vi "Periodic Tasks.vi"(8 "error in":errorcluster) -> ()   [LabVIEW 2016]
doc: "This VI runs in parallel to other tasks. It can contain as many user-defined periodic loops as you need. These can carry out PID or other sorts of timed response."
uses:
  <vilib>/Rock Robotics/WPI/Utilities/WPI_GetSetVariantRefNum.vi
  drive diraction.vi
  <vilib>/Rock Robotics/Network Tables/NT Write Boolean.vi
panel:
  out "rad":bool
  in  "pull":bool
  in  "push":bool
  in  "fire":bool
  in  "gear diraction":bool
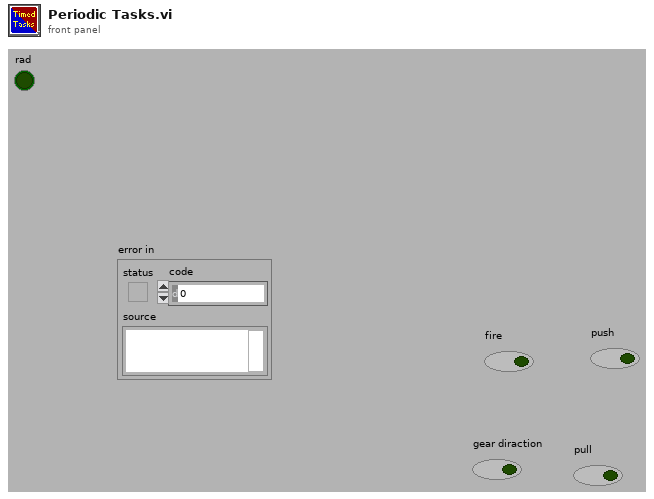
[diagram p1: front panel]
types:
  T1 = typedef "WPI_JoystickDevRef.ctl" = cluster{"Device":T2}
  T2 = typedef "WPI_JoystickDeviceEnum.ctl" = enum16{"USB 0", "USB 1", "USB 2", "USB 3", "USB 4", "USB 5"}
  T3 = cluster{"Buttons[0]":bool, "Buttons[1]":bool, "Buttons[2]":bool, "Buttons[3]":bool, "Buttons[4]":bool, "Buttons[5]":bool, "Buttons[6]":bool, "Buttons[7]":bool, "Buttons[8]":bool}
  T4 = typedef "WPI_MotorControlDeviceRef.ctl" = cluster{"DeviceStatus":errorcluster, "Type":T5, "PWM":cluster{"PWM Channel":T6, "DeadBand":T7}, "CAN":cluster{"Device Number":u8, "SetOutput VI Ref":variant, "GetOutput VI Ref":variant, "Enable VI Ref":variant, "Disable VI Ref":variant, "Data":variant}, "Invert":bool}
  T5 = typedef "WPI_MotorControlType.ctl" = enum16{"PWM", "CAN"}
  T6 = typedef "FPGA_DIOPWMChannel.ctl" = enum8{"PWM 0", "PWM 1", "PWM 2", "PWM 3", "PWM 4", "PWM 5", "PWM 6", "PWM 7", "PWM 8", "PWM 9", "PWM MXP 0", "PWM MXP 1", "PWM MXP 2", "PWM MXP 3", "PWM MXP 4", "PWM MXP 5", "PWM MXP 6", "PWM MXP 7", "PWM MXP 8", "PWM MXP 9", "Invalid"}
  T7 = typedef "WPI_PWMDeadband.ctl" = cluster{"Name":string, "maxPositivePwm":i32, "minPositivePwm":i32, "centerPwm":i32, "maxNegativePwm":i32, "minNegativePwm":i32, "angularRange":u16}
  T8 = typedef "WPI_DigitalInputDevRef.ctl" = cluster{"DevStatus":errorcluster, "DIO Channel":T9}
  T9 = typedef "FPGA_DIOChannel.ctl" = enum8{"DIO 0", "DIO 1", "DIO 2", "DIO 3", "DIO 4", "DIO 5", "DIO 6", "DIO 7", "DIO 8", "DIO 9", "DIO MXP 0", "DIO MXP 1", "DIO MXP 2", "DIO MXP 3", "DIO MXP 4", "DIO MXP 5", "DIO MXP 6", "DIO MXP 7", "DIO MXP 8", "DIO MXP 9", "DIO MXP 10", "DIO MXP 11", "DIO MXP 12", "DIO MXP 13", "DIO MXP 14", "DIO MXP 15", "SPI Port CS1", "SPI Port CS2", "SPI Port CS3", "SPI Port MISO", "SPI Port MOSI", "Invalid"}
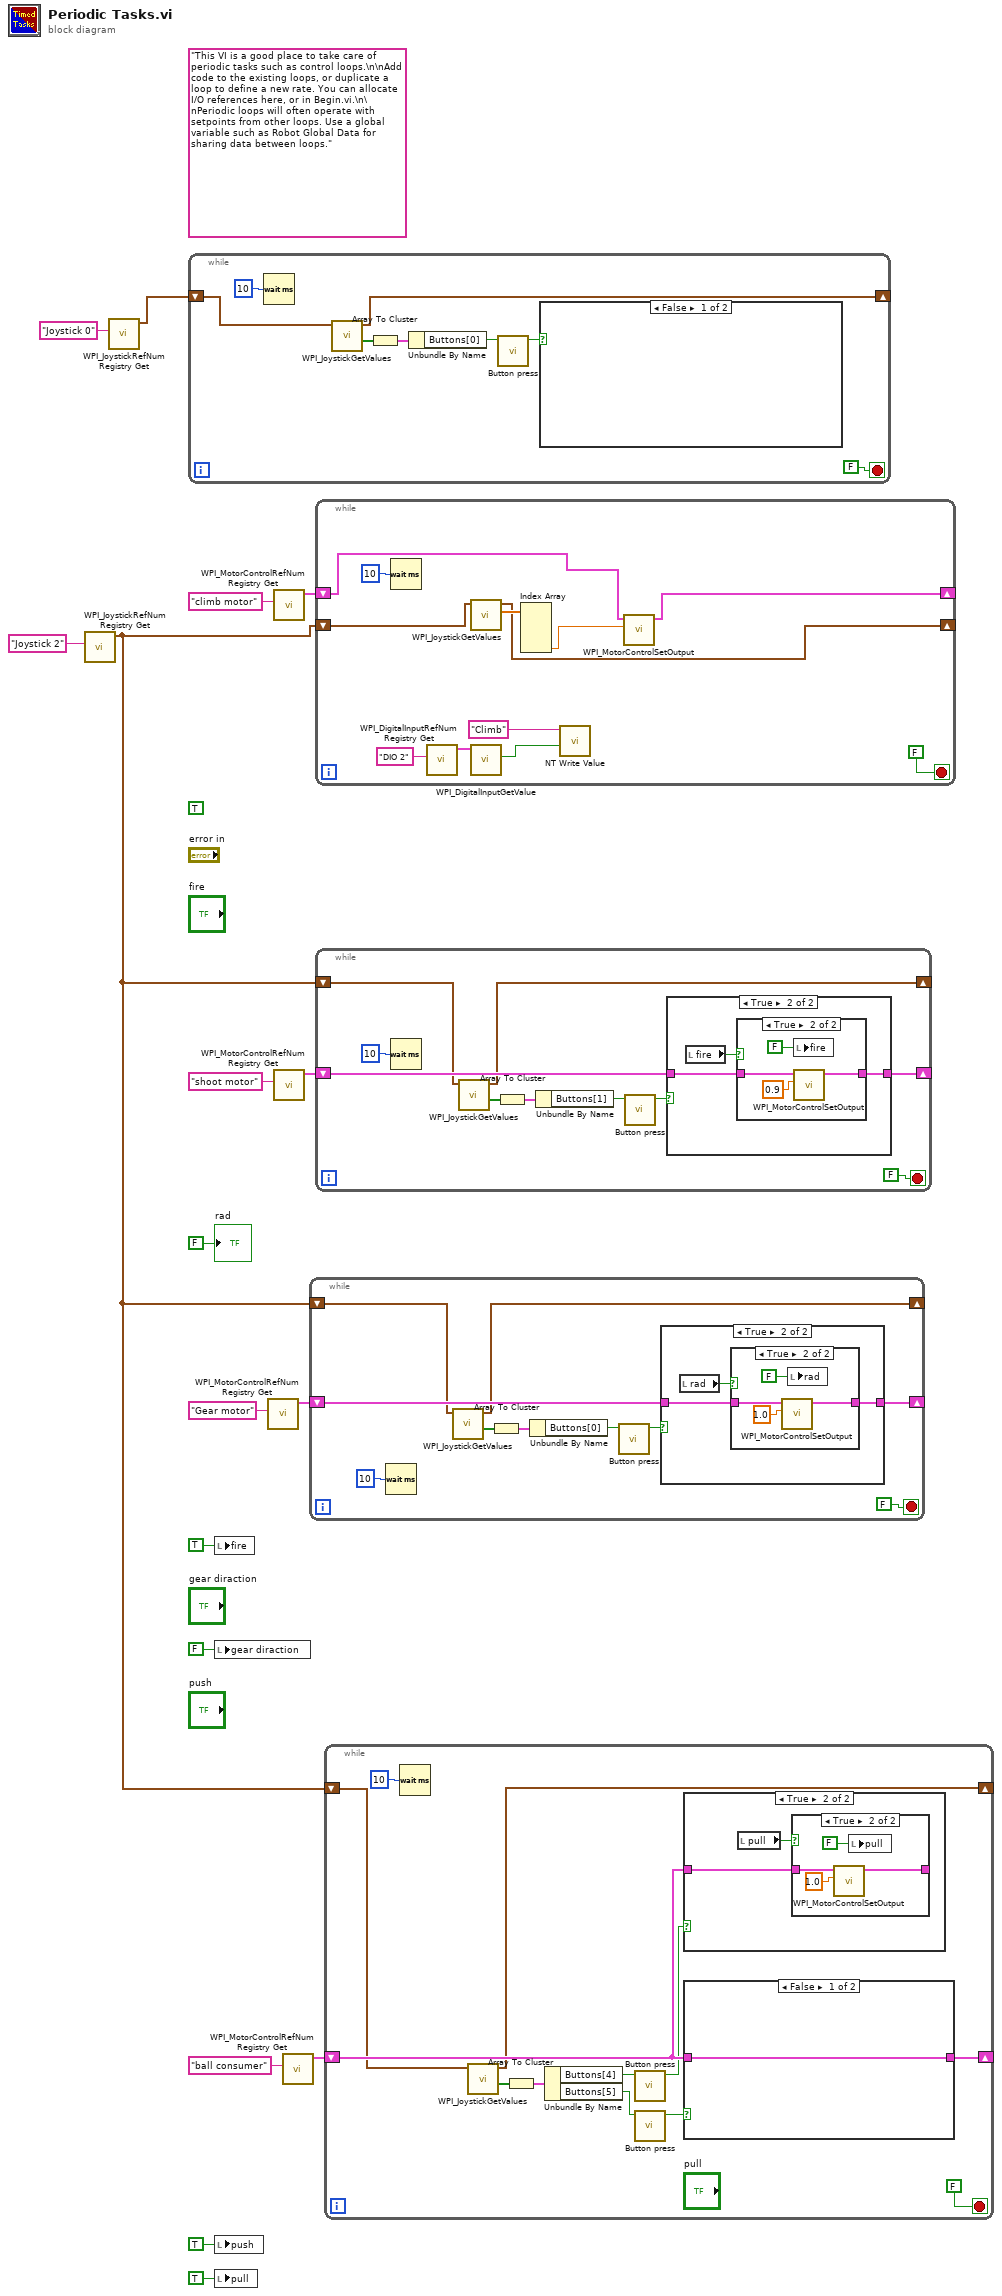
[diagram p0: block diagram]
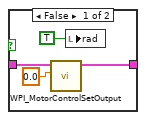
[diagram p3: hidden frame]
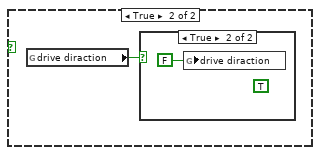
[diagram p4: hidden frame]
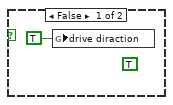
[diagram p5: hidden frame]
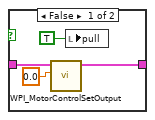
[diagram p7: hidden frame]
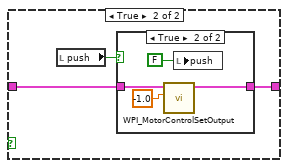
[diagram p8: hidden frame]
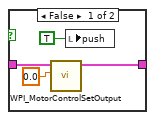
[diagram p9: hidden frame]
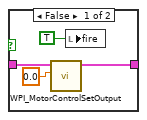
[diagram p11: hidden frame]
diagram:
  (unwired) TRUE ("fire")
  (unwired) "This VI is a good place to take care of periodic tasks such as control loops.\n\nAdd code to the existing loops, or duplicate a loop to define a new rate. You can allocate I/O references here, or in Begin.vi.\n\nPeriodic loops will often operate with setpoints from other loops. Use a global variable such as Robot Global Data for sharing data between loops."
  n1 = call <vilib>:"WPI_JoystickRefNum Registry Get.vi"("refnum name"="Joystick 2") -> ("JoystickDevRef"=w1:T1)  [unwired: 1 in, 9 out]
  n2 = call <vilib>:"WPI_JoystickRefNum Registry Get.vi"("refnum name"="Joystick 0") -> ("JoystickDevRef"=w3:T1)  [unwired: 1 in, 9 out]
  n3 = while {
    shift-right: [w18] -> _
    shift-left: w3 -> [w19]
    stop <- FALSE stop-if-true
    n4 = Wait (ms)(milliseconds to wait=u32 10) -> ()  [unwired: 1 out]
    n5 = call <vilib>:"WPI_JoystickGetValues.vi"("JoystickDevRef"=w19) -> ("Buttons"=w24:bool[], "JoystickDevRef"=w18:T1)  [unwired: 6 in, 3 out]
    n6 = Array To Cluster(array=w24) -> (cluster=w23:T3)
    n7 = Unbundle By Name(w23) -> ("Buttons[0]"=w21:bool)
    n8 = call "Button press.vi"("Boolean"=w21) -> ("Boolean 2"=w20:bool)  [unwired: 10 in]
    n9 = case shown="False" w20 {
      frame False {
      }
      frame True {
        n10 = global read "drive diraction.vi" "drive diraction"() -> (w26:bool)
        n11 = case shown="True" w26 {
          frame False {
            (unwired) TRUE ("fire")
            n12 = global write "drive diraction.vi" "drive diraction"(TRUE ("drive diraction")) -> ()
          }
          frame True {
            (unwired) TRUE ("fire")
            n13 = global write "drive diraction.vi" "drive diraction"(FALSE ("drive diraction")) -> ()
          }
        }
      }
    }
  }
  n14 = local write "fire"(TRUE ("fire")) -> ()
  n15 = local write "gear diraction"(FALSE ("gear diraction")) -> ()
  n16 = local write "push"(TRUE ("push")) -> ()
  n17 = local write "pull"(TRUE ("pull")) -> ()
  n18 = call <vilib>:"WPI_MotorControlRefNum Registry Get.vi"("refnum name"="Gear motor") -> ("MotorControlDevRef"=w6:T4)  [unwired: 9 in, 1 out]
  n19 = call <vilib>:"WPI_MotorControlRefNum Registry Get.vi"("refnum name"="climb motor") -> ("MotorControlDevRef"=w16:T4)  [unwired: 9 in, 1 out]
  n20 = call <vilib>:"WPI_MotorControlRefNum Registry Get.vi"("refnum name"="shoot motor") -> ("MotorControlDevRef"=w15:T4)  [unwired: 9 in, 1 out]
  n21 = call <vilib>:"WPI_MotorControlRefNum Registry Get.vi"("refnum name"="ball consumer") -> ("MotorControlDevRef"=w12:T4)  [unwired: 9 in, 1 out]
  n22 = while {
    shift-right: [w34] -> _
    shift-left: w6 -> [w35]
    shift-right: [w30] -> _
    shift-left: w1 -> [w31]
    stop <- FALSE stop-if-true
    n23 = Wait (ms)(milliseconds to wait=u32 10) -> ()  [unwired: 1 out]
    n24 = call <vilib>:"WPI_JoystickGetValues.vi"("JoystickDevRef"=w31) -> ("Buttons"=w36:bool[], "JoystickDevRef"=w30:T1)  [unwired: 6 in, 3 out]
    n25 = Array To Cluster(array=w36) -> (cluster=w37:T3)
    n26 = Unbundle By Name(w37) -> ("Buttons[0]"=w32:bool)
    n27 = call "Button press.vi"("Boolean"=w32) -> ("Boolean 2"=w33:bool)  [unwired: 10 in]
    n28 = case shown="True" w33 {
      tunnel: w35 -> [w39 w40]
      tunnel: [w39 w41] -> w34
      frame False {
      }
      frame True {
        n29 = local read "rad"() -> (w42:bool)
        n30 = case shown="True" w42 {
          tunnel: [w44 w49] -> w41
          tunnel: w40 -> [w45 w48]
          frame False {
            n31 = call <vilib>:"WPI_MotorControlSetOutput.vi"("Output"=0.0, "MotorControlDevRef"=w45) -> ("MotorControlDevRef"=w44:T4)  [unwired: 7 in, 2 out]
            n32 = local write "rad"(TRUE ("rad")) -> ()
          }
          frame True {
            n33 = call <vilib>:"WPI_MotorControlSetOutput.vi"("Output"=1.0, "MotorControlDevRef"=w48) -> ("MotorControlDevRef"=w49:T4)  [unwired: 7 in, 2 out]
            n34 = local write "rad"(FALSE ("rad")) -> ()
          }
        }
      }
    }
  }
  n35 = while {
    shift-right: [w54] -> _
    shift-left: w16 -> [w55]
    shift-right: [w51] -> _
    shift-left: w1 -> [w52]
    stop <- FALSE stop-if-true
    n36 = Wait (ms)(milliseconds to wait=u32 10) -> ()  [unwired: 1 out]
    n37 = call <vilib>:"WPI_DigitalInputRefNum Registry Get.vi"("refnum name"="DIO 2") -> ("DigitalInputDevRef"=w59:T8)  [unwired: 9 in, 1 out]
    n38 = call <vilib>:"WPI_JoystickGetValues.vi"("JoystickDevRef"=w52) -> ("Axes"=w56:dbl[], "JoystickDevRef"=w51:T1)  [unwired: 6 in, 3 out]
    n39 = call <vilib>:"WPI_DigitalInputGetValue.vi"("DigitalInputDevRef"=w59) -> ("Value"=w58:bool)  [unwired: 8 in, 2 out]
    n40 = Index Array(array=w56) -> (element #4=w53:dbl)  [unwired: 4 in, 3 out]
    n41 = call-poly <vilib>:"NT Write Value.vi"("Boolean"=w58, "Name"="Climb") -> ()  [unwired: 9 in, 1 out]
    n42 = call <vilib>:"WPI_MotorControlSetOutput.vi"("Output"=w53, "MotorControlDevRef"=w55) -> ("MotorControlDevRef"=w54:T4)  [unwired: 7 in, 2 out]
  }
  n43 = while {
    shift-right: [w69] -> _
    shift-left: w15 -> [w68]
    shift-right: [w63] -> _
    shift-left: w1 -> [w64]
    stop <- FALSE stop-if-true
    n44 = Wait (ms)(milliseconds to wait=u32 10) -> ()  [unwired: 1 out]
    n45 = call <vilib>:"WPI_JoystickGetValues.vi"("JoystickDevRef"=w64) -> ("Buttons"=w71:bool[], "JoystickDevRef"=w63:T1)  [unwired: 6 in, 3 out]
    n46 = Array To Cluster(array=w71) -> (cluster=w70:T3)
    n47 = Unbundle By Name(w70) -> ("Buttons[1]"=w66:bool)
    n48 = call "Button press.vi"("Boolean"=w66) -> ("Boolean 2"=w65:bool)  [unwired: 10 in]
    n49 = case shown="True" w65 {
      tunnel: [w73 w76] -> w69
      tunnel: w68 -> [w73 w75]
      frame False {
      }
      frame True {
        n50 = local read "fire"() -> (w74:bool)
        n51 = case shown="True" w74 {
          tunnel: [w79 w83] -> w76
          tunnel: w75 -> [w80 w84]
          frame False {
            n52 = call <vilib>:"WPI_MotorControlSetOutput.vi"("Output"=0.0, "MotorControlDevRef"=w80) -> ("MotorControlDevRef"=w79:T4)  [unwired: 7 in, 2 out]
            n53 = local write "fire"(TRUE ("fire")) -> ()
          }
          frame True {
            n54 = local write "fire"(FALSE ("fire")) -> ()
            n55 = call <vilib>:"WPI_MotorControlSetOutput.vi"("Output"=0.9, "MotorControlDevRef"=w84) -> ("MotorControlDevRef"=w83:T4)  [unwired: 7 in, 2 out]
          }
        }
      }
    }
  }
  n56 = while {
    shift-right: [w93] -> _
    shift-left: w12 -> [w91]
    shift-right: [w85] -> _
    shift-left: w1 -> [w86]
    stop <- FALSE stop-if-true
    n57 = Wait (ms)(milliseconds to wait=u32 10) -> ()  [unwired: 1 out]
    n58 = call <vilib>:"WPI_JoystickGetValues.vi"("JoystickDevRef"=w86) -> ("Buttons"=w95:bool[], "JoystickDevRef"=w85:T1)  [unwired: 6 in, 3 out]
    n59 = Array To Cluster(array=w95) -> (cluster=w94:T3)
    n60 = Unbundle By Name(w94) -> ("Buttons[4]"=w89:bool, "Buttons[5]"=w90:bool)
    n61 = call "Button press.vi"("Boolean"=w89) -> ("Boolean 2"=w87:bool)  [unwired: 10 in]
    n62 = call "Button press.vi"("Boolean"=w90) -> ("Boolean 2"=w88:bool)  [unwired: 10 in]
    n63 = case shown="True" w87 {
      tunnel: w91 -> [_ w98]
      frame False {
      }
      frame True {
        n64 = local read "pull"() -> (w97:bool)
        n65 = case shown="True" w97 {
          tunnel: [w101 w104] -> _
          tunnel: w98 -> [w102 w105]
          frame False {
            n66 = call <vilib>:"WPI_MotorControlSetOutput.vi"("Output"=0.0, "MotorControlDevRef"=w102) -> ("MotorControlDevRef"=w101:T4)  [unwired: 7 in, 2 out]
            n67 = local write "pull"(TRUE ("pull")) -> ()
          }
          frame True {
            n68 = call <vilib>:"WPI_MotorControlSetOutput.vi"("Output"=1.0, "MotorControlDevRef"=w105) -> ("MotorControlDevRef"=w104:T4)  [unwired: 7 in, 2 out]
            n69 = local write "pull"(FALSE ("pull")) -> ()
          }
        }
      }
    }
    n70 = case shown="False" w88 {
      tunnel: [w107 w110] -> w93
      tunnel: w91 -> [w107 w109]
      frame False {
      }
      frame True {
        n71 = local read "push"() -> (w108:bool)
        n72 = case shown="True" w108 {
          tunnel: [w114 w116] -> w110
          tunnel: w109 -> [w113 w117]
          frame False {
            n73 = call <vilib>:"WPI_MotorControlSetOutput.vi"("Output"=0.0, "MotorControlDevRef"=w113) -> ("MotorControlDevRef"=w114:T4)  [unwired: 7 in, 2 out]
            n74 = local write "push"(TRUE ("push")) -> ()
          }
          frame True {
            n75 = call <vilib>:"WPI_MotorControlSetOutput.vi"("Output"=-1.0, "MotorControlDevRef"=w117) -> ("MotorControlDevRef"=w116:T4)  [unwired: 7 in, 2 out]
            n76 = local write "push"(FALSE ("push")) -> ()
          }
        }
      }
    }
  }
  "rad" <- FALSE ("Boolean")
